vi "DDSSequence.vi"() -> ()   [LabVIEW 2016]
panel:
  in  "Freqeuncy (MHz)":dbl[][](array[numeric])=[[1.0, 2.0, 2.0, 1.0, 0.5, 0.0]]
  in  "Power":dbl[][](array[numeric])=[[1.0, 0.0, 0.5, 0.0, 1.0, 0.0]]
  out "Instruction String Slot 2":string="dds 0 reset\rdcp 0 spi:CFR2=0x1000080\rdcp 0 spi:STP0=0x418937\rdcp 0 wait::BNC_IN_A_RISING\rdcp 0 update:u\rdcp 0 spi:STP0=0x3FFF000000418937\rdcp 0 wait:0h:\rdcp 0 update:u\r\rdcp 0 spi:STP0=0x83126F\rdcp 0 wait:62500h:\rdcp 0 update:u\r\rdcp 0 spi:STP0=0x3FFF00000083126F\rdcp 0 wait:31250h:\rdcp 0 update:u\r\rdcp 0 spi:STP0=0x418937\rdcp 0 wait:62500h:\rdcp 0 update:u\r\rdcp 0 spi:DRL=0xFFFC000000000000\rdcp 0 spi:DRSS=0x28F5C29028F5C29\rdcp 0 spi:DRR=0x1F401F4\rdcp 0 spi:CFR2=0x280080\rdcp 0 wait:62500h:\rdcp 0 update:u+d\rdcp 0 wait:125000h:\rdcp 0 update:-d\rdcp 0 spi:CFR2=0x1200080\rdcp 0 spi:STP0=0x418937\rdcp 0 wait:62500h:\rdcp 0 update:u\rdcp 0 start\rdds 1 reset\rdcp 1 spi:CFR2=0x1000080\rdcp 1 spi:STP0=0x418937\rdcp 1 wait::BNC_IN_A_RISING\rdcp 1 update:u\rdcp 1 spi:STP0=0x3FFF000000418937\rdcp 1 wait:0h:\rdcp 1 update:u\r\rdcp 1 spi:STP0=0x83126F\rdcp 1 wait:62500h:\rdcp 1 update:u\r\rdcp 1 spi:STP0=0x200000000083126F\rdcp 1 wait:31250h:\rdcp 1 update:u\r\rdcp 1 spi:STP0=0x418937\rdcp 1 wait:62500h:\rdcp 1 update:u\r\rdcp 1 spi:DRL=0xFFFC000000000000\rdcp 1 spi:DRSS=0x28F5C29028F5C29\rdcp 1 spi:DRR=0x1F401F4\rdcp 1 spi:CFR2=0x280080\rdcp 1 wait:62500h:\rdcp 1 update:u+d\rdcp 1 wait:125000h:\rdcp 1 update:-d\rdcp 1 spi:CFR2=0x1200080\rdcp 1 spi:STP0=0x418937\rdcp 1 wait:62500h:\rdcp 1 update:u\rdcp 1 start\r\r"
  in  "Freqeuncy (MHz)":dbl[][](array[numeric])=[[1.0, 2.0, 2.0, 1.0, 0.5, 0.0]]
  in  "Power":dbl[][](array[numeric])=[[1.0, 0.0, 1.0, 0.0, 1.0, 0.0]]
  out "return count 2":u32
  out "error out 2":errorcluster={"status"=TRUE, "code"=-1073807343, "source"="Property Node (arg 1) in VISA Configure Serial Port (Instr).vi->FlexDDS-NG_USB_VISA_Open.vi->DDSSequence.vi"}
  out "read buffer 2":string
  in  "Freqeuncy (MHz)":dbl[][](array[numeric])=[[1.0, 2.0, 2.0, 1.0, 0.5, 0.0]]
  in  "Power":dbl[][](array[numeric])=[[1.0, 0.0, 0.5, 0.0, 1.0, 0.0]]
  out "Instruction String Slot 1":string="dds 0 reset\rdcp 0 spi:CFR2=0x1000080\rdcp 0 spi:STP0=0x418937\rdcp 0 wait::BNC_IN_A_RISING\rdcp 0 update:u\rdcp 0 spi:STP0=0x3FFF000000418937\rdcp 0 wait:0h:\rdcp 0 update:u\r\rdcp 0 spi:STP0=0x83126F\rdcp 0 wait:62500h:\rdcp 0 update:u\r\rdcp 0 spi:STP0=0x3FFF00000083126F\rdcp 0 wait:31250h:\rdcp 0 update:u\r\rdcp 0 spi:STP0=0x418937\rdcp 0 wait:62500h:\rdcp 0 update:u\r\rdcp 0 spi:DRL=0xFFFC000000000000\rdcp 0 spi:DRSS=0x28F5C29028F5C29\rdcp 0 spi:DRR=0x1F401F4\rdcp 0 spi:CFR2=0x280080\rdcp 0 wait:62500h:\rdcp 0 update:u+d\rdcp 0 wait:125000h:\rdcp 0 update:-d\rdcp 0 spi:CFR2=0x1200080\rdcp 0 spi:STP0=0x418937\rdcp 0 wait:62500h:\rdcp 0 update:u\rdcp 0 start\rdds 1 reset\rdcp 1 spi:CFR2=0x1000080\rdcp 1 spi:STP0=0x418937\rdcp 1 wait::BNC_IN_A_RISING\rdcp 1 update:u\rdcp 1 spi:STP0=0x3FFF000000418937\rdcp 1 wait:0h:\rdcp 1 update:u\r\rdcp 1 spi:STP0=0x83126F\rdcp 1 wait:62500h:\rdcp 1 update:u\r\rdcp 1 spi:STP0=0x200000000083126F\rdcp 1 wait:31250h:\rdcp 1 update:u\r\rdcp 1 spi:STP0=0x418937\rdcp 1 wait:62500h:\rdcp 1 update:u\r\rdcp 1 spi:DRL=0xFFFC000000000000\rdcp 1 spi:DRSS=0x28F5C29028F5C29\rdcp 1 spi:DRR=0x1F401F4\rdcp 1 spi:CFR2=0x280080\rdcp 1 wait:62500h:\rdcp 1 update:u+d\rdcp 1 wait:125000h:\rdcp 1 update:-d\rdcp 1 spi:CFR2=0x1200080\rdcp 1 spi:STP0=0x418937\rdcp 1 wait:62500h:\rdcp 1 update:u\rdcp 1 start\r\r"
  in  "No of  active time blocks":dbl=4.0
  in  "Freqeuncy (MHz)":dbl[][](array[numeric])=[[1.0, 2.0, 2.0, 1.0, 0.5, 0.0]]
  in  "Duration (ms)":dbl[][](array[numeric])=[[0.5, 0.25, 0.5, 1.0, 2.0, 1.0]]
  in  "Power":dbl[][](array[numeric])=[[1.0, 0.0, 1.0, 0.0, 1.0, 0.0]]
  out "return count":u32=1275
  out "error out":errorcluster={"status"=TRUE, "code"=-1073807339, "source"="VISA Read in DDSSequence.vi"}
  out "read buffer":string
  # "Laser Cooling"
  # "Repumper"
  # "DDS 3"
  # "DDS 4"
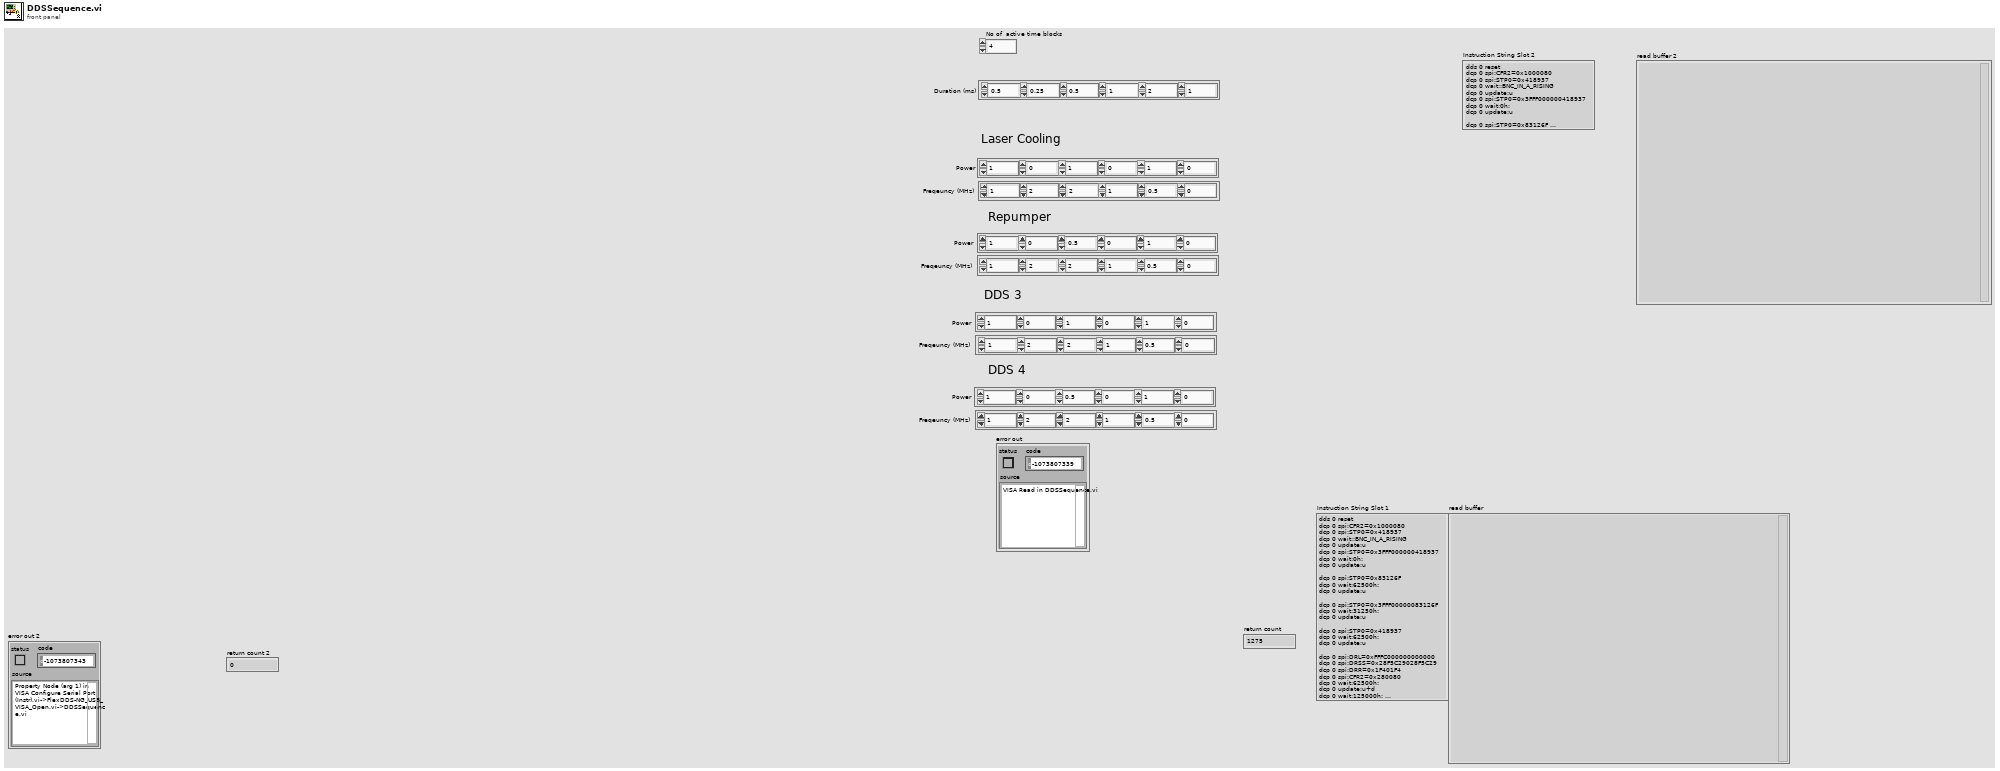
[diagram p1: front panel]
types:
  T1 = enum32{"Channel 0", "Channel 1", "Both channels"}
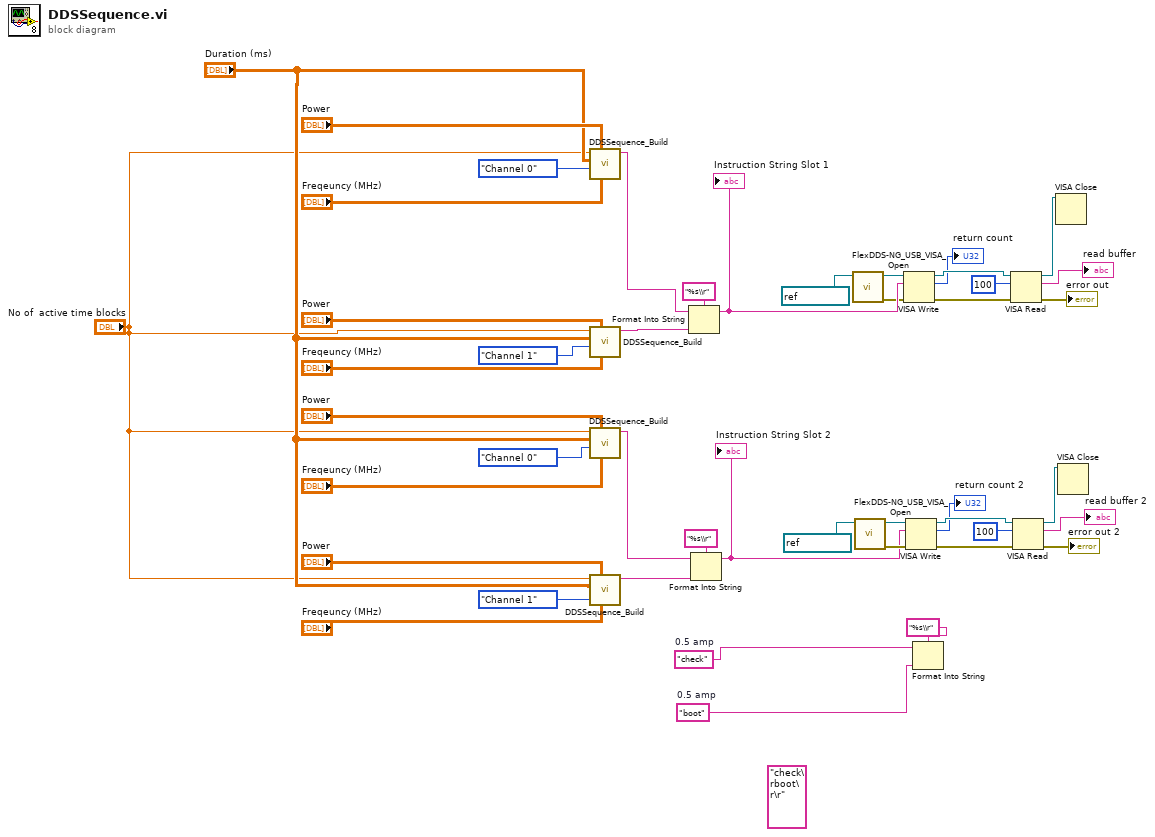
[diagram p0: block diagram]
diagram:
  (unwired) "check\rboot\r\r" ("appended instruction string 5")
  w12 = "boot"  # 0.5 amp
  w13 = "check"  # 0.5 amp
  n1 = call "DDSSequence_Build.vi"("Freqeuncy (MHz)"="Freqeuncy (MHz)", "Power"="Power", "Channels"=T1."Channel 0", "Duration (ms)"="Duration (ms)", "No of  active time blocks"="No of  active time blocks") -> ("appended instruction string"=w27:string)  [unwired: 6 in]
  n2 = call "DDSSequence_Build.vi"("Freqeuncy (MHz)"="Freqeuncy (MHz)", "Power"="Power", "Channels"=T1."Channel 1", "Duration (ms)"="Duration (ms)", "No of  active time blocks"="No of  active time blocks") -> ("appended instruction string"=w36:string)  [unwired: 6 in]
  n3 = call "DDSSequence_Build.vi"("Freqeuncy (MHz)"="Freqeuncy (MHz)", "Power"="Power", "Channels"=T1."Channel 0", "Duration (ms)"="Duration (ms)", "No of  active time blocks"="No of  active time blocks") -> ("appended instruction string"=w1:string)  [unwired: 6 in]
  n4 = call "DDSSequence_Build.vi"("Freqeuncy (MHz)"="Freqeuncy (MHz)", "Power"="Power", "Channels"=T1."Channel 1", "Duration (ms)"="Duration (ms)", "No of  active time blocks"="No of  active time blocks") -> ("appended instruction string"=w29:string)  [unwired: 6 in]
  n5 = Format Into String(format string="%s\\r", initial string=w27, w36) -> (resulting string=w26:string)  [unwired: 1 in, 1 out]
  "Instruction String Slot 1" <- w26
  n6 = Format Into String(format string="%s\\r", initial string=w1, w29) -> (resulting string=w11:string)  [unwired: 1 in, 1 out]
  "Instruction String Slot 2" <- w11
  n7 = call "FlexDDS-NG_USB_VISA_Open.vi"("FlexDDS-NG USB VISA resource name (COM)"=refnum<visa-resource-name> "COM11") -> ("error out"=w3:errorcluster, "FlexDDS-NG USB VISA resource name out"=w4:refnum<visa-resource-name>)  [unwired: 9 in]
  n8 = call "FlexDDS-NG_USB_VISA_Open.vi"("FlexDDS-NG USB VISA resource name (COM)"=refnum<visa-resource-name> "COM12") -> ("error out"=w16:errorcluster, "FlexDDS-NG USB VISA resource name out"=w17:refnum<visa-resource-name>)  [unwired: 9 in]
  n9 = VISA Write(VISA resource name=w4, write buffer=w26, error in (no error)=w3) -> (VISA resource name out=w8:refnum<visa-resource-name>, return count=→"return count":u32, error out=w6:errorcluster)
  n10 = VISA Write(VISA resource name=w17, write buffer=w11, error in (no error)=w16) -> (VISA resource name out=w21:refnum<visa-resource-name>, return count=→"return count 2":u32, error out=w19:errorcluster)
  n11 = Format Into String(format string="%s\\r", initial string=w13, w12) -> ()  [unwired: 1 in, 2 out]
  n12 = VISA Read(VISA resource name=w8, byte count=u32 100, error in (no error)=w6) -> (VISA resource name out=w15:refnum<visa-resource-name>, read buffer=→"read buffer":string, error out=→"error out":errorcluster)  [unwired: 1 out]
  n13 = VISA Read(VISA resource name=w21, byte count=u32 100, error in (no error)=w19) -> (VISA resource name out=w24:refnum<visa-resource-name>, read buffer=→"read buffer 2":string, error out=→"error out 2":errorcluster)  [unwired: 1 out]
  n14 = VISA Close(VISA resource name=w15) -> ()  [unwired: 1 in, 1 out]
  n15 = VISA Close(VISA resource name=w24) -> ()  [unwired: 1 in, 1 out]
